vi "5492_DoYouEvenLift.vi"(0 "MotorControlDevRef":T1={"DeviceStatus"={"status"=FALSE, "code"=0, "source"=""}, "Type"=enum."PWM", "PWM"={"PWM Channel"=enum."Invalid", "DeadBand"={"Name"="", "maxPositivePwm"=0, "minPositivePwm"=0, "centerPwm"=0, "maxNegativePwm"=0, "minNegativePwm"=0, "angularRange"=0}}, "CAN"={"Device Number"=0, "SetOutput VI Ref"=variant(enum8{"Percent VBus", "Current", "Speed", "Position", "Voltage"} enum."Percent VBus"), "GetOutput VI Ref"=variant(refnum<k1> refnum), "Enable VI Ref"=variant(dbl 12.0), "Disable VI Ref"=variant(enum8{"Percent VBus", "Speed", "Position", "Slave", "Unchanged / Invalid", "Voltage Compensation", "Current", "Motion Profile"} enum."Percent VBus"), "Data"=variant}, "Invert"=FALSE, "DIO PWM"={"PWM \"Enable\" Channel"=enum."Invalid", "DIOChannel"=enum."Invalid", "PWM Rate"=0.0}}, 5 "Hi?":bool, 7 "Low?":bool, 9 "Collect?":bool, 11 "Setting":string) -> (4 "MotorControlDevRef 2":T1={"DeviceStatus"={"status"=FALSE, "code"=0, "source"=""}, "Type"=enum."PWM", "PWM"={"PWM Channel"=enum."Invalid", "DeadBand"={"Name"="", "maxPositivePwm"=0, "minPositivePwm"=0, "centerPwm"=0, "maxNegativePwm"=0, "minNegativePwm"=0, "angularRange"=0}}, "CAN"={"Device Number"=0, "SetOutput VI Ref"=variant(enum8{"Percent VBus", "Current", "Speed", "Position", "Voltage"} enum."Percent VBus"), "GetOutput VI Ref"=variant(refnum<k1> refnum), "Enable VI Ref"=variant(dbl 12.0), "Disable VI Ref"=variant(enum8{"Percent VBus", "Speed", "Position", "Slave", "Unchanged / Invalid", "Voltage Compensation", "Current", "Motion Profile"} enum."Percent VBus"), "Data"=variant}, "Invert"=FALSE, "DIO PWM"={"PWM \"Enable\" Channel"=enum."Invalid", "DIOChannel"=enum."Invalid", "PWM Rate"=0.0}}, 15 "Setting but Out":string)   [LabVIEW 2017]
uses:
  <vilib>/Rock Robotics/WPI/MotorControl/WPI_MotorControlDeviceRef.ctl
  <vilib>/Rock Robotics/WPI/MotorControl/WPI_MotorControlType.ctl
  <vilib>/Rock Robotics/SystemInterfaces/DIO/FPGA_DIOPWMChannel.ctl
  <vilib>/Rock Robotics/WPI/PWM/WPI_PWMDeadband.ctl
  <vilib>/Rock Robotics/SystemInterfaces/DIO/FPGA_DIOChannel.ctl
  Public/Documents/Cross The Road Electronics/Phoenix-LabVIEW/Motor Controller/Controls/CTRE_Phoenix_MotorControl_ControlMode.ctl
  5492_LiftButtons.vi
  <vilib>/Rock Robotics/WPI/MotorControl/WPI_MotorControlSafetyCheck.vi
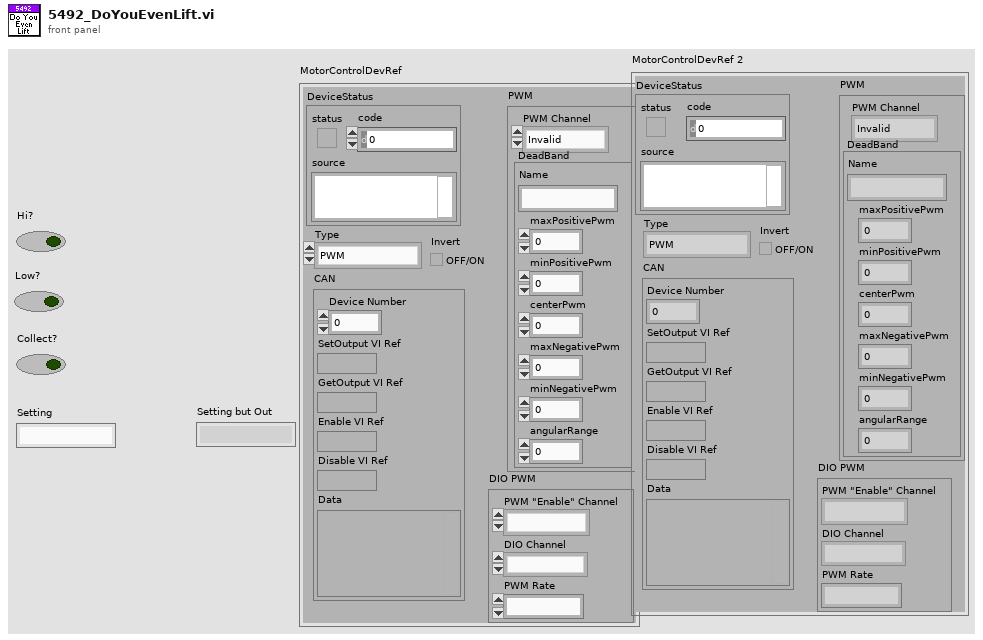
[diagram p1: front panel]
types:
  T1 = typedef "WPI_MotorControlDeviceRef.ctl" = cluster{"DeviceStatus":errorcluster, "Type":T2, "PWM":cluster{"PWM Channel":T3, "DeadBand":T4}, "CAN":cluster{"Device Number":u8, "SetOutput VI Ref":variant, "GetOutput VI Ref":variant, "Enable VI Ref":variant, "Disable VI Ref":variant, "Data":variant}, "Invert":bool, "DIO PWM":cluster{"PWM \"Enable\" Channel":T3, "DIOChannel":T5, "PWM Rate":dbl}}
  T2 = typedef "WPI_MotorControlType.ctl" = enum16{"PWM", "CAN", "DIO PWM"}
  T3 = typedef "FPGA_DIOPWMChannel.ctl" = enum8{"PWM 0", "PWM 1", "PWM 2", "PWM 3", "PWM 4", "PWM 5", "PWM 6", "PWM 7", "PWM 8", "PWM 9", "PWM MXP 0", "PWM MXP 1", "PWM MXP 2", "PWM MXP 3", "PWM MXP 4", "PWM MXP 5", "PWM MXP 6", "PWM MXP 7", "PWM MXP 8", "PWM MXP 9", "Invalid"}
  T4 = typedef "WPI_PWMDeadband.ctl" = cluster{"Name":string, "maxPositivePwm":i32, "minPositivePwm":i32, "centerPwm":i32, "maxNegativePwm":i32, "minNegativePwm":i32, "angularRange":u16}
  T5 = typedef "FPGA_DIOChannel.ctl" = enum8{"DIO 0", "DIO 1", "DIO 2", "DIO 3", "DIO 4", "DIO 5", "DIO 6", "DIO 7", "DIO 8", "DIO 9", "DIO MXP 0", "DIO MXP 1", "DIO MXP 2", "DIO MXP 3", "DIO MXP 4", "DIO MXP 5", "DIO MXP 6", "DIO MXP 7", "DIO MXP 8", "DIO MXP 9", "DIO MXP 10", "DIO MXP 11", "DIO MXP 12", "DIO MXP 13", "DIO MXP 14", "DIO MXP 15", "SPI Port CS1", "SPI Port CS2", "SPI Port CS3", "SPI Port MISO", "SPI Port MOSI", "Invalid"}
  T6 = typedef "CTRE_Phoenix_MotorControl_ControlMode.ctl" = u16
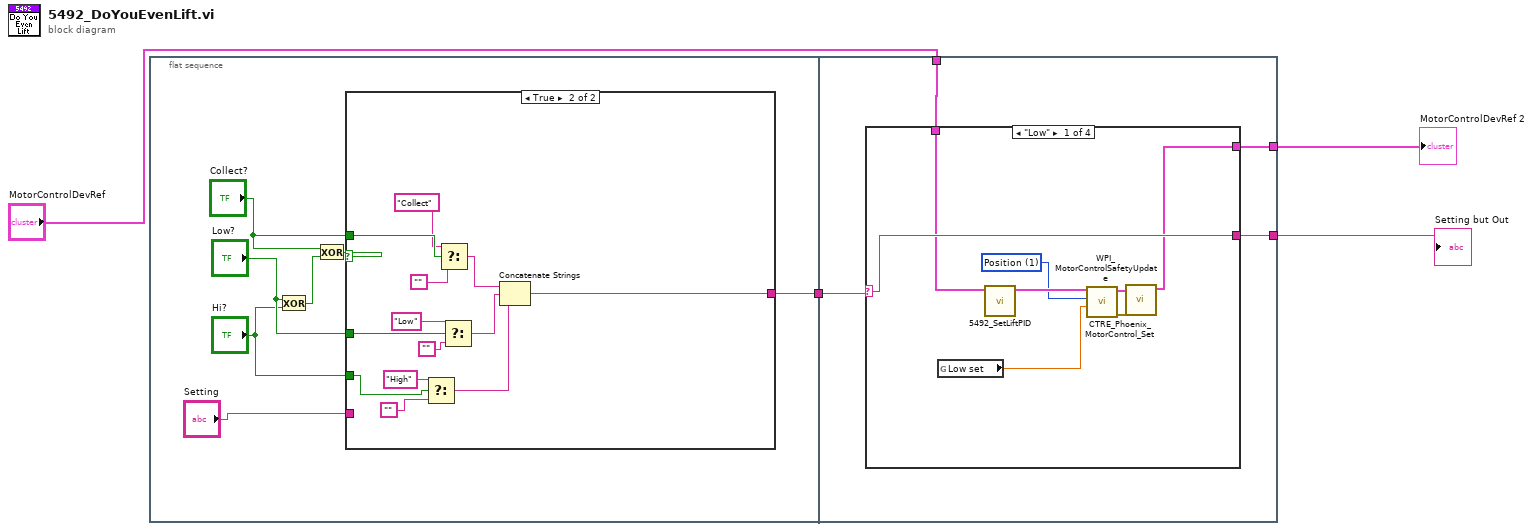
[diagram p0: block diagram]
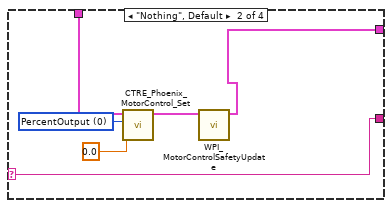
[diagram p3: hidden frame]
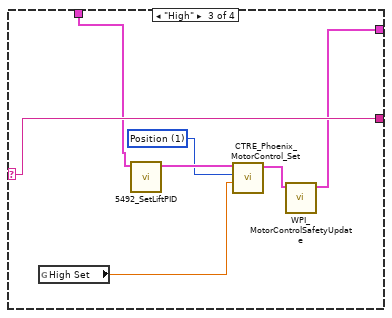
[diagram p4: hidden frame]
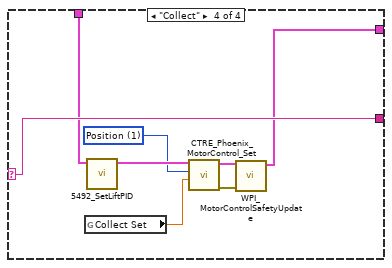
[diagram p5: hidden frame]
diagram:
  n1 = flat-sequence {
    tunnel: [w5] -> w4
    tunnel: w4 -> [w29]
    tunnel: [w28] -> w3
    tunnel: "MotorControlDevRef" -> [w27]
    tunnel: [w26] -> w1
    frame #0 {
      n2 = Exclusive Or(1:"Hi?", 2:"Low?") -> (0:w11:bool)
      n3 = Exclusive Or(1:w11, 2:"Collect?") -> (0:w10:bool)
      n4 = case shown="True" w10 {
        tunnel: "Collect?" -> [_ w23]
        tunnel: "Low?" -> [_ w21]
        tunnel: "Setting" -> [w12 _]
        tunnel: "Hi?" -> [_ w15]
        tunnel: [w12 w13] -> w5
        frame False {
        }
        frame True {
          n5 = Select(t="High", s=w15, f="") -> (s? t:f=w14:string)
          n6 = Select(t="Collect", s=w23, f="") -> (s? t:f=w24:string)
          n7 = Select(t="Low", s=w21, f="") -> (s? t:f=w18:string)
          n8 = Concatenate Strings(w24, w18, w14) -> (w13:string)
        }
      }
    }
    frame #1 {
      n9 = case shown="\"Low\"" w29 {
        selector: w29 -> [w35 w43 w48 w56]
        tunnel: [w35 w43 w48 w56] -> w28
        tunnel: w27 -> [w31 w40 w47 w52]
        tunnel: [w32 w42 w45 w53] -> w26
        frame "Low" {
          w36 = T6 1 items=["PercentOutput"=0, "Position"=1, "Velocity"=2, "Current"=3, "Follower"=5, "MotionProfile"=6, "MotionMagic"=7, "MotionMagicArc"=8, "MotionProfileArc"=10, "Disabled"=15] ("Control Mode")
          n10 = global read "5492_LiftButtons.vi" "Low set"() -> (w30:dbl)
          n11 = call "5492_SetLiftPID.vi"("PhoenixMotorControlDevRef 2"=w31) -> ("PhoenixMotorControlDevRef"=w37:T1)  [unwired: 9 in, 1 out]
          n12 = call "CTRE_Phoenix_MotorControl_Set.vi"("Output"=w30, "Control Mode"=w36, "PhoenixMotorControlDevRef"=w37) -> ("error out"=w34:errorcluster, "PhoenixMotorControlDevRef"=w33:T1)  [unwired: 7 in]
          n13 = call <vilib>:"WPI_MotorControlSafetyUpdate.vi"("error in (no error)"=w34, "MotorControlDevRef"=w33) -> ("MotorControlDevRef"=w32:T1)  [unwired: 9 out]
        }
        frame "Nothing", Default {
          w39 = T6 0 items=["PercentOutput"=0, "Position"=1, "Velocity"=2, "Current"=3, "Follower"=5, "MotionProfile"=6, "MotionMagic"=7, "MotionMagicArc"=8, "MotionProfileArc"=10, "Disabled"=15] ("Control Mode")
          n14 = call "CTRE_Phoenix_MotorControl_Set.vi"("Output"=0.0, "Control Mode"=w39, "PhoenixMotorControlDevRef"=w40) -> ("PhoenixMotorControlDevRef"=w41:T1)  [unwired: 7 in, 1 out]
          n15 = call <vilib>:"WPI_MotorControlSafetyUpdate.vi"("MotorControlDevRef"=w41) -> ("MotorControlDevRef"=w42:T1)  [unwired: 1 in, 9 out]
        }
        frame "High" {
          w49 = T6 1 items=["PercentOutput"=0, "Position"=1, "Velocity"=2, "Current"=3, "Follower"=5, "MotionProfile"=6, "MotionMagic"=7, "MotionMagicArc"=8, "MotionProfileArc"=10, "Disabled"=15] ("Control Mode")
          n16 = global read "5492_LiftButtons.vi" "High Set"() -> (w44:dbl)
          n17 = call "5492_SetLiftPID.vi"("PhoenixMotorControlDevRef 2"=w47) -> ("PhoenixMotorControlDevRef"=w50:T1)  [unwired: 9 in, 1 out]
          n18 = call "CTRE_Phoenix_MotorControl_Set.vi"("Output"=w44, "Control Mode"=w49, "PhoenixMotorControlDevRef"=w50) -> ("PhoenixMotorControlDevRef"=w46:T1)  [unwired: 7 in, 1 out]
          n19 = call <vilib>:"WPI_MotorControlSafetyUpdate.vi"("MotorControlDevRef"=w46) -> ("MotorControlDevRef"=w45:T1)  [unwired: 1 in, 9 out]
        }
        frame "Collect" {
          w57 = T6 1 items=["PercentOutput"=0, "Position"=1, "Velocity"=2, "Current"=3, "Follower"=5, "MotionProfile"=6, "MotionMagic"=7, "MotionMagicArc"=8, "MotionProfileArc"=10, "Disabled"=15] ("Control Mode")
          n20 = global read "5492_LiftButtons.vi" "Collect Set"() -> (w51:dbl)
          n21 = call "5492_SetLiftPID.vi"("PhoenixMotorControlDevRef 2"=w52) -> ("PhoenixMotorControlDevRef"=w58:T1)  [unwired: 9 in, 1 out]
          n22 = call "CTRE_Phoenix_MotorControl_Set.vi"("Output"=w51, "Control Mode"=w57, "PhoenixMotorControlDevRef"=w58) -> ("error out"=w55:errorcluster, "PhoenixMotorControlDevRef"=w54:T1)  [unwired: 7 in]
          n23 = call <vilib>:"WPI_MotorControlSafetyUpdate.vi"("error in (no error)"=w55, "MotorControlDevRef"=w54) -> ("MotorControlDevRef"=w53:T1)  [unwired: 9 out]
        }
      }
    }
  }
  "Setting but Out" <- w3
  "MotorControlDevRef 2" <- w1
